vi "Replace Outside VIs.vi"(8 "error in (no error)":errorcluster, 9 "Shared directory":path, 10 "Non-Library VI[]":string[](array[string]), 11 "Measurement directory":path) -> (0 "error out":errorcluster)   [LabVIEW 2021]
uses:
  <vilib>/Utility/traverseref.llb/TRef TravTarget.ctl
  <vilib>/Utility/traverseref.llb/VI Scripting - Traverse.lvlib
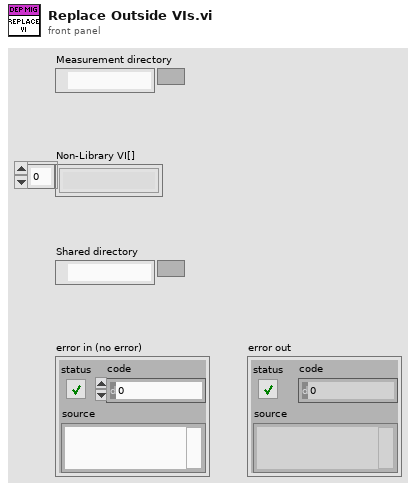
[diagram p1: front panel]
types:
  T1 = typedef "TRef TravTarget.ctl" = enum16{"FP", "BD", "Other"}
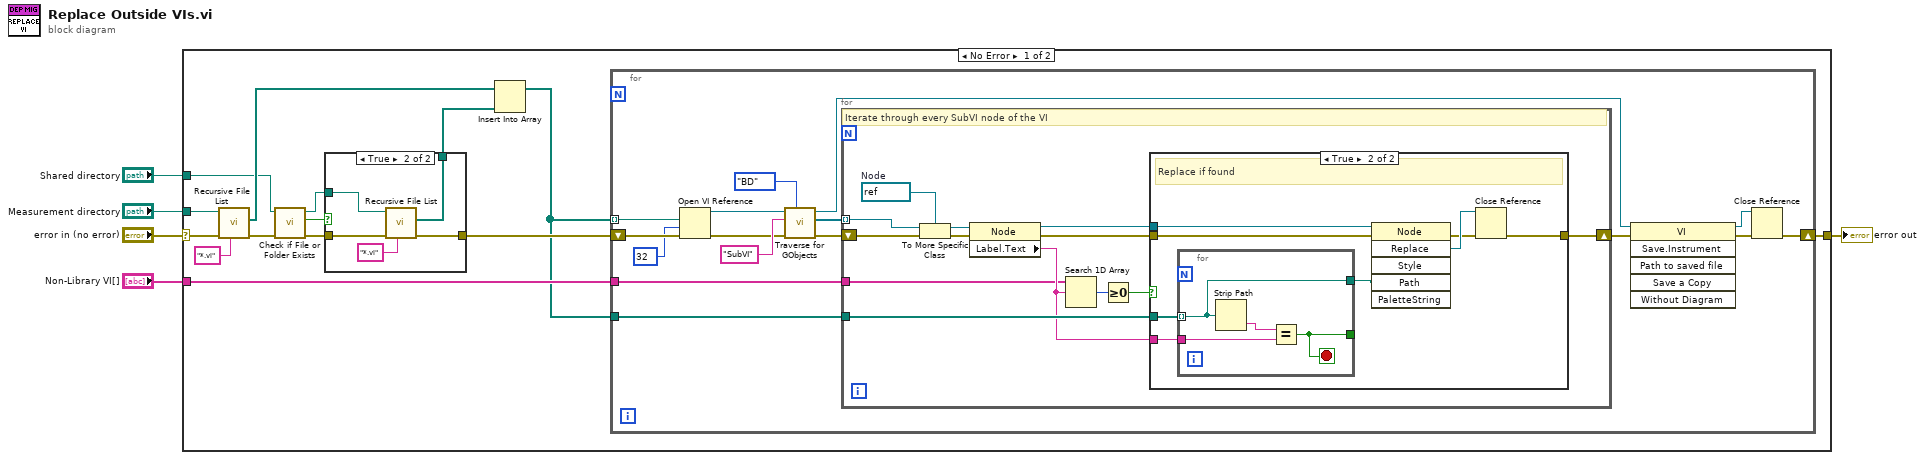
[diagram p0: block diagram]
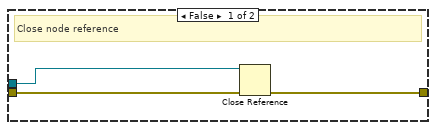
[diagram p3: hidden frame]
diagram:
  n1 = case shown="No Error" "error in (no error)" {
    selector: "error in (no error)" -> [w18 w70]
    tunnel: "Non-Library VI[]" -> [w19 _]
    tunnel: "Measurement directory" -> [w17 _]
    tunnel: [w15 w70] -> w2
    tunnel: "Shared directory" -> [w8 _]
    frame No Error {
      n2 = call <vilib>:"Recursive File List.vi"("pattern"="*.vi", "error in (no error)"=w18, "Folder Path"=w17) -> ("error out"=w14:errorcluster, "All Files in Dir"=w12:path[])  [unwired: 4 in, 3 out]
      n3 = call <vilib>:"Check if File or Folder Exists.vi"("error in (no error)"=w14, "path"=w8) -> ("error out"=w9:errorcluster, "file or folder exists?"=w6:bool, "dup path"=w7:path)  [unwired: 7 in]
      n4 = case shown="True" w6 {
        tunnel: w9 -> [w20 w24]
        tunnel: [w20 w23] -> w13
        tunnel: [_ w22] -> w11
        tunnel: w7 -> [_ w21]
        frame False {
        }
        frame True {
          n5 = call <vilib>:"Recursive File List.vi"("pattern"="*.vi", "error in (no error)"=w24, "Folder Path"=w21) -> ("error out"=w23:errorcluster, "All Files in Dir"=w22:path[])  [unwired: 4 in, 3 out]
        }
      }
      n6 = Insert Into Array(array=w12, new element=w11) -> (w10:path[])  [unwired: 1 in]
      n7 = for {
        tunnel: w10 -> [w40]
        tunnel: w19 -> [w39]
        tunnel: w10 -> [w31] mode=indexing
        shift-right: [w32] -> w15
        shift-left: w13 -> [w34]
        n8 = Open VI Reference(vi path=w31, options=32, error in (no error)=w34) -> (vi reference=w30:refnum<vi>, error out=w33:errorcluster)  [unwired: 3 in]
        n9 = call <vilib>:"Traverse for GObjects.vi"("Traverse Target"=TRef_TravTarget."BD", "error in (no error)"=w33, "Class Name"="SubVI" ("name/order"), "VI Refnum"=w30) -> ("error out"=w38:errorcluster, "References"=w41:refnum<vi>[], "dup VI Refnum"=w28:refnum<vi>)  [unwired: 4 in, 1 out]
        n10 = for {
          tunnel: w41 -> [w54] mode=indexing
          shift-right: [w49] -> w37
          shift-left: w38 -> [w53]
          tunnel: w39 -> [w42]
          tunnel: w40 -> [w47]
          w44 = refnum<vi> refnum  # Node
          # "Iterate through every SubVI node of the VI"
          n11 = To More Specific Class(target class=w44, reference=w54, error in=w53) -> (specific class reference=w45:refnum<vi>, error out=w43:errorcluster)
          n12 = property class="Node"(reference=w45, error in=w43) -> (reference out=w50:refnum<vi>, error out=w51:errorcluster, "Label.Text"=w46:string)
          n13 = Search 1D Array(1D array=w42, element=w46) -> (index of element=w52:i32)  [unwired: 1 in]
          n14 = Greater Or Equal To 0?(x=w52) -> (x >= 0?=w48:bool)
          n15 = case shown="True" w48 {
            tunnel: w51 -> [w57 w65]
            tunnel: w50 -> [w56 w64]
            tunnel: [w55 w58] -> w49
            tunnel: w47 -> [_ w63]
            tunnel: w46 -> [_ w62]
            frame False {
              # "Close node reference"
              n16 = Close Reference(reference=w56, error in (no error)=w57) -> (error out=w55:errorcluster)
            }
            frame True {
              # "Replace if found"
              n17 = for {
                tunnel: w63 -> [w67] mode=indexing
                tunnel: w62 -> [w68]
                tunnel: [w67] -> w61
                tunnel: [w66] -> _
                stop <- w66 stop-if-true
                n18 = Strip Path(path=w67) -> (name=w69:string)  [unwired: 1 out]
                n19 = Equal?(x=w69, y=w68) -> (x = y?=w66:bool)
              }
              n20 = invoke class="Node" method="Replace"(reference=w64, error in=w65, "Path"=w61) -> (error out=w59:errorcluster, "Replace"=w60:refnum<vi>)  [unwired: 3 in, 4 out]
              n21 = Close Reference(reference=w60, error in (no error)=w59) -> (error out=w58:errorcluster)
            }
          }
        }
        n22 = invoke class="VI" method="Save.Instrument"(reference=w28, error in=w37) -> (reference out=w27:refnum<vi>, error out=w29:errorcluster)  [unwired: 4 in, 4 out]
        n23 = Close Reference(reference=w27, error in (no error)=w29) -> (error out=w32:errorcluster)
      }
    }
    frame Error {
    }
  }
  "error out" <- w2
